vi "FileIO-Write Anything.vi"(7 "Prompt?":bool, 8 "error in (no error)":errorcluster, 9 "Section Name":string, 10 "Anything":variant, 11 "Settings file":path) -> (0 "error out":errorcluster, 1 "Saved?":bool, 3 "Path out":path)   [LabVIEW 2020]
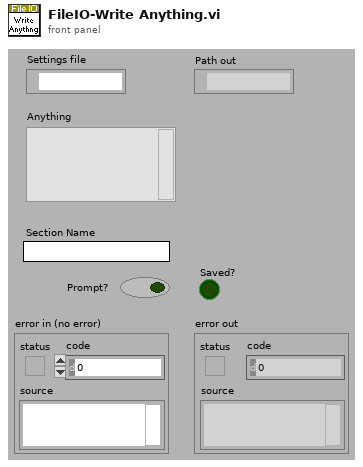
[diagram p1: front panel]
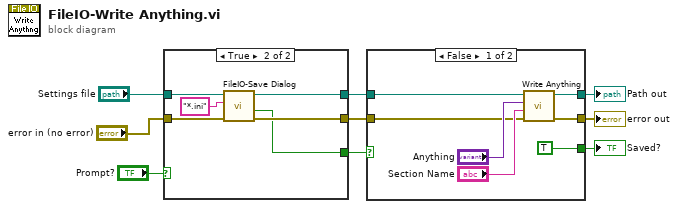
[diagram p0: block diagram]
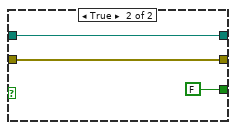
[diagram p2: hidden frame]
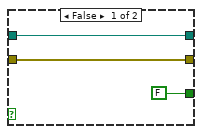
[diagram p3: hidden frame]
diagram:
  n1 = case shown="True" "Prompt?" {
    tunnel: "Settings file" -> [w12 w18]
    tunnel: "error in (no error)" -> [w11 w16]
    tunnel: [w11 w15] -> w5
    tunnel: [w12 w14] -> w4
    tunnel: [FALSE ("cancelled") w13] -> w6
    frame False {
    }
    frame True {
      n2 = call "FileIO-Save Dialog.vi"("error in"=w16, "pattern (all files)"="*.ini", "Start path"=w18) -> ("error out"=w15:errorcluster, "cancelled"=w13:bool, "selected path"=w14:path)  [unwired: 6 in]
    }
  }
  n3 = case shown="False" w6 {
    tunnel: w5 -> [w23 w27]
    tunnel: w4 -> [w22 w28]
    tunnel: [w21 w28] -> w1
    tunnel: [w20 w27] -> w3
    tunnel: [TRUE FALSE] -> w2
    frame False {
      n4 = call "Write Anything.vi"("Error In"=w23, "Section Name (Name of \"Anything\")"="Section Name", "Anything"="Anything", "Path (dialog)"=w22) -> ("Error Out"=w20:errorcluster, "Path out"=w21:path)  [unwired: 6 in]
    }
    frame True {
    }
  }
  "error out" <- w3
  "Saved?" <- w2
  "Path out" <- w1
